vi "Address Remote Terminal.vi"(7 "Virtual Memory Unit in":refnum<class "Virtual Memory Unit.lvclass">, 8 "error in (no error)":errorcluster, 11 "Remote Terminal in":refnum<class "Remote Terminal.lvclass">) -> (0 "error out":errorcluster, 3 "Remote Terminal out":refnum<class "Remote Terminal.lvclass">, 5 "Virtual Memory Unit out":refnum<class "Virtual Memory Unit.lvclass">)   [LabVIEW 2020, in "BCI-1553 API.lvlib" / "Remote Terminal.lvclass"]
doc: "Sets the address for this Remote Terminal and ensures that the container for the address has odd parity."
uses:
  Remote Terminal.lvclass
  Dependencies/Virtual Memory Unit/Virtual Memory Unit.lvclass
  Remote Terminal.lvclass/Remote Terminal.ctl
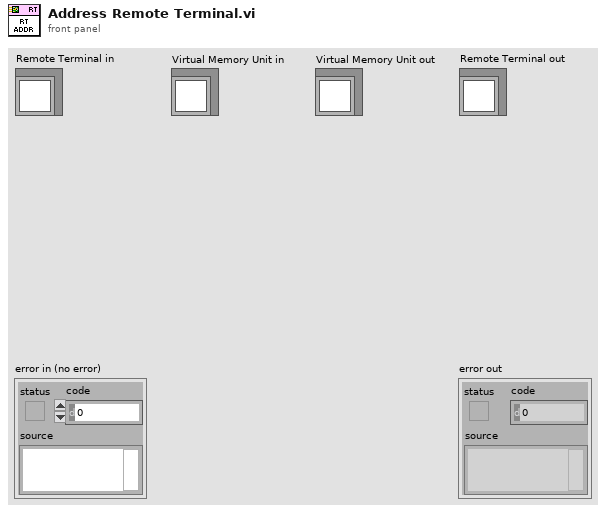
[diagram p1: front panel]
types:
  T1 = typedef "BCI-1553 API.lvlib/Command Terminal Address.ctl" = enum16{"0", "1", "2", "3", "4", "5", "6", "7", "8", "9", "10", "11", "12", "13", "14", "15", "16", "17", "18", "19", "20", "21", "22", "23", "24", "25", "26", "27", "28", "29", "30", "Broadcast"}
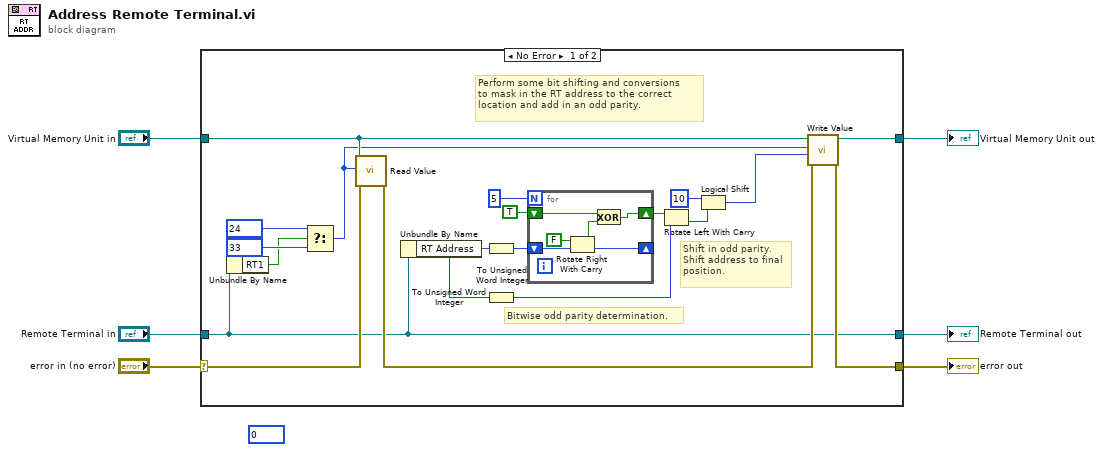
[diagram p0: block diagram]
diagram:
  (unwired) 0 ("Address")
  n1 = case shown="No Error" "error in (no error)" {
    selector: "error in (no error)" -> [w22 w34]
    tunnel: [w18 w34] -> w5
    tunnel: [w16 w33] -> w3
    tunnel: "Remote Terminal in" -> [w16 w33]
    tunnel: "Virtual Memory Unit in" -> [w21 w32]
    tunnel: [w20 w32] -> w1
    frame No Error {
      # "Shift in odd parity.\nShift address to final\nposition."
      # "Bitwise odd parity determination."
      # "Perform some bit shifting and conversions\nto mask in the RT address to the correct\nlocation and add in an odd parity."
      n2 = Unbundle By Name(w16) -> ("RT1"=w23:bool)
      n3 = Select(t=24 ("Address"), s=w23, f=33 ("Address")) -> (s? t:f=w17:i32)
      n4 = call "Read Value.vi"("error in (no error)"=w22, "Index"=w17, "Virtual Memory Unit in"=w21) -> ("error out"=w19:errorcluster)  [unwired: 7 in, 1 out]
      n5 = Unbundle By Name(w16) -> ("RT Address"=w10:T1)
      n6 = To Unsigned Word Integer(number=w10) -> (unsigned 16bit integer=w7:u16)
      n7 = To Unsigned Word Integer(number=w10) -> (unsigned 16bit integer=w8:u16)
      n8 = for {
        N: 5 -> [_]
        shift-right: [w30] -> _
        shift-left: w7 -> [w31]
        shift-right: [w26] -> w12
        shift-left: TRUE -> [w27]
        n9 = Rotate Right With Carry(2:w31, 3:FALSE ("carry")) -> (0:w30:u16, 1:w28:bool)
        n10 = Exclusive Or(1:w28, 2:w27) -> (0:w26:bool)
      }
      n11 = Rotate Left With Carry(2:w8, 3:w12) -> (0:w11:u16)  [unwired: 1 out]
      n12 = Logical Shift(y=i16 10, x=w11) -> (x << y=w9:u16)
      n13 = call "Write Value.vi"("error in (no error)"=w19, "Value"=w9, "Index"=w17, "Virtual Memory Unit in"=w21) -> ("error out"=w18:errorcluster, "Virtual Memory Unit out"=w20:refnum<class "Virtual Memory Unit.lvclass">)  [unwired: 6 in]
    }
    frame Error {
    }
  }
  "error out" <- w5
  "Remote Terminal out" <- w3
  "Virtual Memory Unit out" <- w1
